vi "Set CAN Bit Rate.vi"(6 "New Baud Rate":u16(ring) items=["1 Mbit/s"=1000, "800 kbit/s"=800, "500 kbit/s"=500, "250 kbit/s"=250, "125 kbit/s"=125, "50 kbit/s"=50, "20 kbit/s"=20], 7 "timeout (1s)":dbl=1.0 min=0.0, 8 "error in (no error)":errorcluster, 11 "SDO object in":refnum<k20>) -> (0 "error out":errorcluster, 1 "completion code":u32, 3 "SDO object out":refnum<k20>)   [LabVIEW 2016]
uses:
  <vilib>/CANopenLib/CANOPEN.llb/CANopen SDO Write [U16].vi
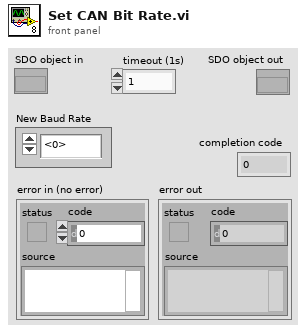
[diagram p1: front panel]
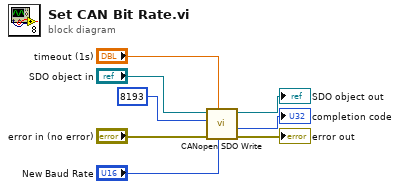
[diagram p0: block diagram]
diagram:
  n1 = call-poly <vilib>:"CANopen SDO Write.vi"("U16 data"="New Baud Rate", "timeout (1s)"="timeout (1s)", "error in (no error)"="error in (no error)", "object index"=u16 8193, "SDO object in"="SDO object in") -> ("error out"=→"error out":errorcluster, "completion code"=→"completion code":u32, "SDO object out"=→"SDO object out":refnum<k20>)  [unwired: 4 in]
